vi "Get Data.vi"(8 "error in (no error)":errorcluster, 11 "Tree Data Folder in":refnum<class "Tree Data Folder.lvclass">) -> (0 "error out":errorcluster, 3 "Tree Data Folder out":refnum<class "Tree Data Folder.lvclass">)   [LabVIEW 2022 SP3, in "Tree Data Folder.lvclass"]
uses:
  Tree Data Folder.lvclass
  C:/Users/User/Desktop/Bussiness/Tricorn Re/Mandelbrot 4.0/General Library V2/Ancestor Class/Front Panel Container/Tree/Tree Data/Tree Data.lvclass
  C:/Users/User/Desktop/Bussiness/Tricorn Re/Mandelbrot 4.0/General Library V2/Ancestor Class/Front Panel Container/Tree/Composite Tree Data/Composite Tree Data.lvclass
  Tree Data Folder.lvclass/Tree Data Folder.ctl
  Tree Data File/Tree Data File.lvclass/Tree Data File.ctl
  Composite Tree Data/Composite Tree Data.lvclass/Composite Tree Data.ctl
  Public Data/Write Folder Path.vi
  Tree Data File/Public Data/Write File Path.vi
  Composite Tree Data/Protected Data/Write Sub Nodes.vi
  Protected Data/Write Files.vi
  Tree Data File/Tree Data File.lvclass
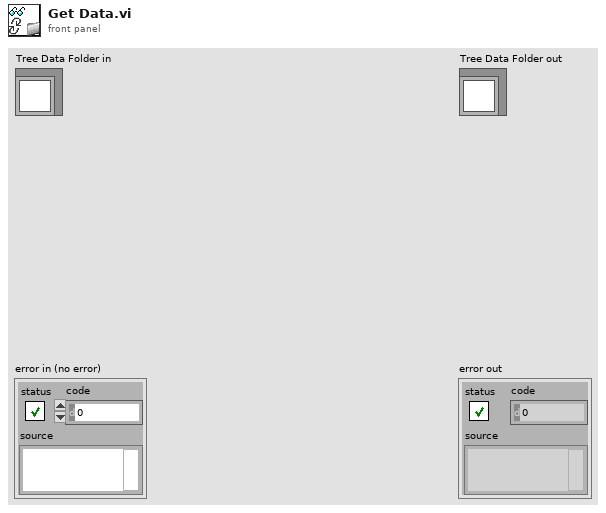
[diagram p1: front panel]
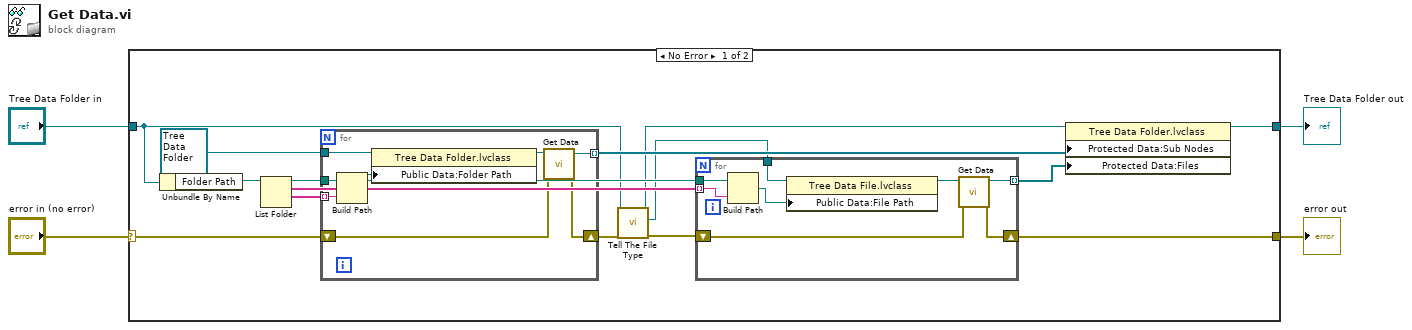
[diagram p0: block diagram]
diagram:
  n1 = case shown="No Error" "error in (no error)" {
    selector: "error in (no error)" -> [w16 w37]
    tunnel: [w12 w37] -> w3
    tunnel: [w13 w36] -> w1
    tunnel: "Tree Data Folder in" -> [w7 w36]
    frame No Error {
      n2 = Unbundle By Name(w7) -> ("Folder Path"=w10:path)
      n3 = List Folder(path=w10) -> (path out=w18:path, filenames=w19:string[], folder names=w17:string[])  [unwired: 3 in, 1 out]
      n4 = for {
        tunnel: w18 -> [w27]
        tunnel: w17 -> [w26] mode=indexing
        shift-right: [w23] -> w9
        shift-left: w16 -> [w24]
        tunnel: refnum<class "Tree Data Folder.lvclass"> refnum ("Tree Data Folder.lvclass") -> [w21]
        tunnel: [w25] -> w14 mode=indexing
        n5 = Build Path(base path=w27, name or relative path=w26) -> (appended path=w20:path)
        n6 = property class="Tree Data Folder.lvclass"(reference=w21, "Public Data:Folder Path"=w20) -> (reference out=w22:refnum<class "Tree Data Folder.lvclass">)  [unwired: 1 in, 1 out]
        n7 = call-dynamic "Get Data.vi"("error in (no error)"=w24, "Tree Data Folder in"=w22) -> ("error out"=w23:errorcluster, "Tree Data Folder out"=w25:refnum<class "Tree Data Folder.lvclass">)  [unwired: 8 in]
      }
      n8 = call-dynamic "Tell The File Type.vi"("error in (no error)"=w9, "Tree Data Folder in"=w7) -> ("error out"=w8:errorcluster, "File Type Out"=w5:refnum<class "Tree Data File.lvclass">, "Tree Data Folder out"=w6:refnum<class "Tree Data Folder.lvclass">)  [unwired: 7 in]
      n9 = for {
        tunnel: w19 -> [w34] mode=indexing
        tunnel: w18 -> [w35]
        shift-right: [w31] -> w12
        shift-left: w8 -> [w32]
        tunnel: [w33] -> w11 mode=indexing
        tunnel: w5 -> [w30]
        n10 = Build Path(base path=w35, name or relative path=w34) -> (appended path=w28:path)
        n11 = property class="Tree Data File.lvclass"(reference=w30, "Public Data:File Path"=w28) -> (reference out=w29:refnum<class "Tree Data File.lvclass">)  [unwired: 1 in, 1 out]
        n12 = call-dynamic "Get Data.vi"("error in (no error)"=w32, "Tree Data File in"=w29) -> ("error out"=w31:errorcluster, "Tree Data File out"=w33:refnum<class "Tree Data File.lvclass">)  [unwired: 8 in]
      }
      n13 = property class="Tree Data Folder.lvclass"(reference=w6, "Protected Data:Sub Nodes"=w14, "Protected Data:Files"=w11) -> (reference out=w13:refnum<class "Tree Data Folder.lvclass">)  [unwired: 1 in, 1 out]
    }
    frame Error {
    }
  }
  "error out" <- w3
  "Tree Data Folder out" <- w1
